vi "VCS Get Velocity Is Averaged.vi"(8 "error in (no error)":errorcluster, 11 "axis in":cluster{"keyHandle":u32, "nodeId":u16}={"keyHandle"=0, "nodeId"=1}) -> (0 "error out":errorcluster, 2 "velocityIsAveraged":i32, 3 "axis out":cluster{"keyHandle":u32, "nodeId":u16}={"keyHandle"=0, "nodeId"=1})   [LabVIEW 2010]
doc: "<B>VCS Get Velocity Is Averaged</B> reads the velocity actual averaged value."
uses:
  Resources/EposCmd.dll
  Resources/EposCmd64.dll
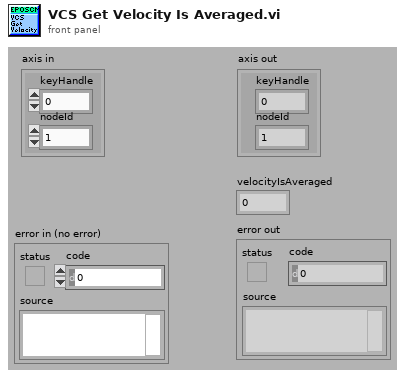
[diagram p1: front panel]
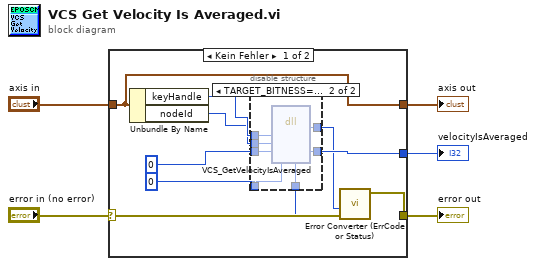
[diagram p0: block diagram]
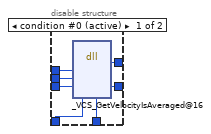
[diagram p2: hidden frame]
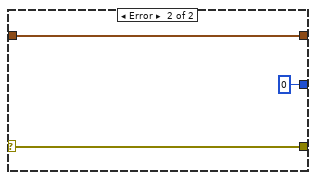
[diagram p3: hidden frame]
diagram:
  n1 = case shown="Kein Fehler" "error in (no error)" {
    selector: "error in (no error)" -> [w13 w32]
    tunnel: [w12 w32] -> w4
    tunnel: [w15 0 ("pVelocityIs")] -> w3
    tunnel: "axis in" -> [w7 w31]
    tunnel: [w7 w31] -> w1
    frame No Error {
      n2 = Unbundle By Name(w7) -> ("keyHandle"=w10:u32, "nodeId"=w9:u16)
      n3 = disable-structure shown="TARGET_BITNESS==64" {
        disable-tunnel: [w22 w29] -> w15
        disable-tunnel: u32 0 ("pErrorCode") -> [w21 w28]
        disable-tunnel: [w20 w27] -> w11
        disable-tunnel: w10 -> [w19 w26]
        disable-tunnel: w9 -> [w18 w25]
        disable-tunnel: 0 ("pVelocityIs") -> [w17 w24]
        disable-tunnel: [w16 w23] -> w6
        frame condition #0 (active) {
          n4 = dll-call lib="C:/Sources/LabView/maxon EPOS/Resources/EposCmd.*" fn="_VCS_GetVelocityIsAveraged@16" ("EposCmd.dll:_VCS_GetVelocityIs@16")("KeyHandle"=w19, "NodeId"=w18, "pVelocityIsAveraged"=w17, "pErrorCode"=w21) -> (w16:i32, "pVelocityIsAveraged"=w22:i32, "pErrorCode"=w20:u32)  [unwired: 5 in, 2 out]
        }
        frame condition #1 {
          n5 = dll-call lib="C:/setup/Resources/EposCmd64.*" fn="VCS_GetVelocityIsAveraged" ("EposCmd.dll:_VCS_GetVelocityIs@16")("KeyHandle"=w26, "NodeId"=w25, "pVelocityIsAveraged"=w24, "pErrorCode"=w28) -> ("Rückgabetyp"=w23:i32, "pVelocityIsAveraged"=w29:i32, "pErrorCode"=w27:u32)  [unwired: 5 in, 2 out]
        }
      }
      n6 = call "Error Converter (ErrCode or Status).vi"("error code"=w11, "return type"=w6, "error in (no error)"=w13) -> ("error out"=w12:errorcluster)  [unwired: 7 in]
    }
    frame Error {
    }
  }
  "velocityIsAveraged" <- w3
  "error out" <- w4
  "axis out" <- w1
